vi "EOL CAN_Get_Motor_DTC's (2).vi"(10 "DTC Select Array":bool[](array[boolean])=[FALSE, FALSE, FALSE, FALSE, FALSE, FALSE, FALSE, FALSE, FALSE, FALSE, FALSE, FALSE, FALSE, FALSE, FALSE, FALSE, FALSE, FALSE, FALSE, FALSE], 11 "NetworkObjHandle":u32) -> (0 "DTC's Set":bool, 1 "DTC String":string, 2 "No. of DTC's":i32, 3 "Response Good?":bool, 5 "TxRx Data":string[][](array[string]))   [LabVIEW 2012]
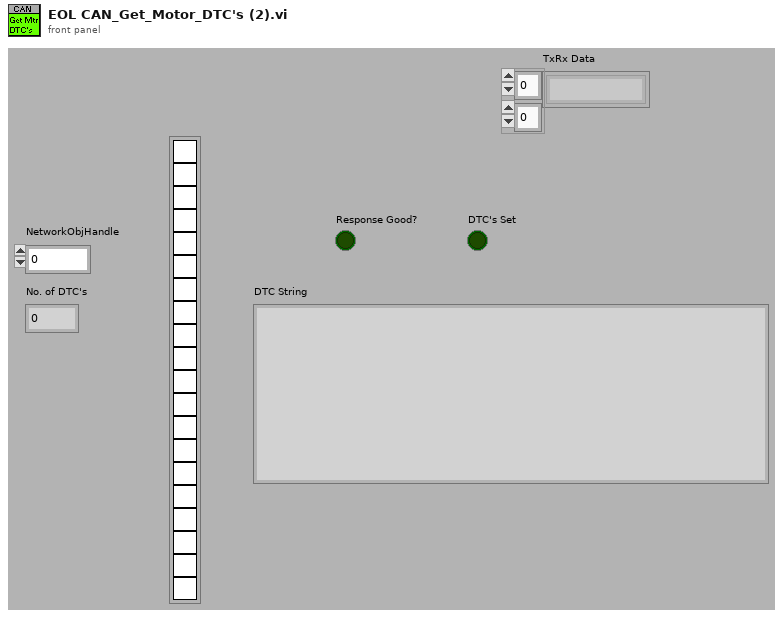
[diagram p1: front panel]
types:
  T1 = cluster{"Retry Counter":i32, "Array 1":u8[], "Array 21":u8[], "Array 22":u8[], "Array 23":u8[], "DTC's Array":u8[][], "No. of DTC's":i32, "Response Good?":bool, "TxRx Data":string[][]}
  T2 = typedef "xobjhandle.ctl" = u32
  T3 = typedef "CanFrameTimed.ctl" = cluster{"Timestamp":dbl, "ArbitrationId":u32, "IsRemote":u8, "DataLength":u8, "Data":u8[]}
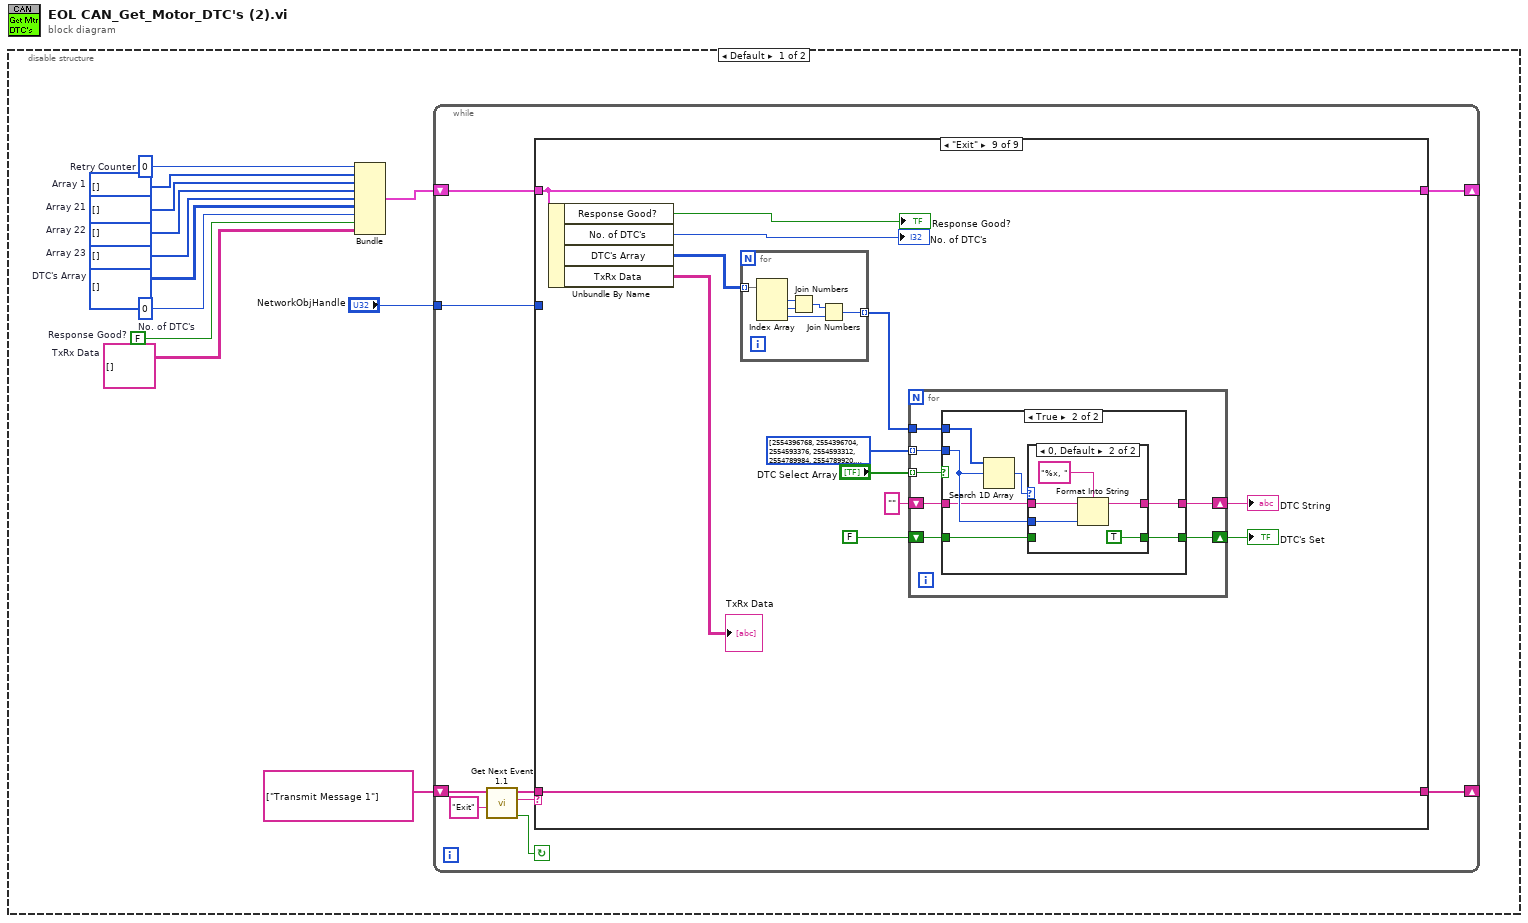
[diagram p0: block diagram]
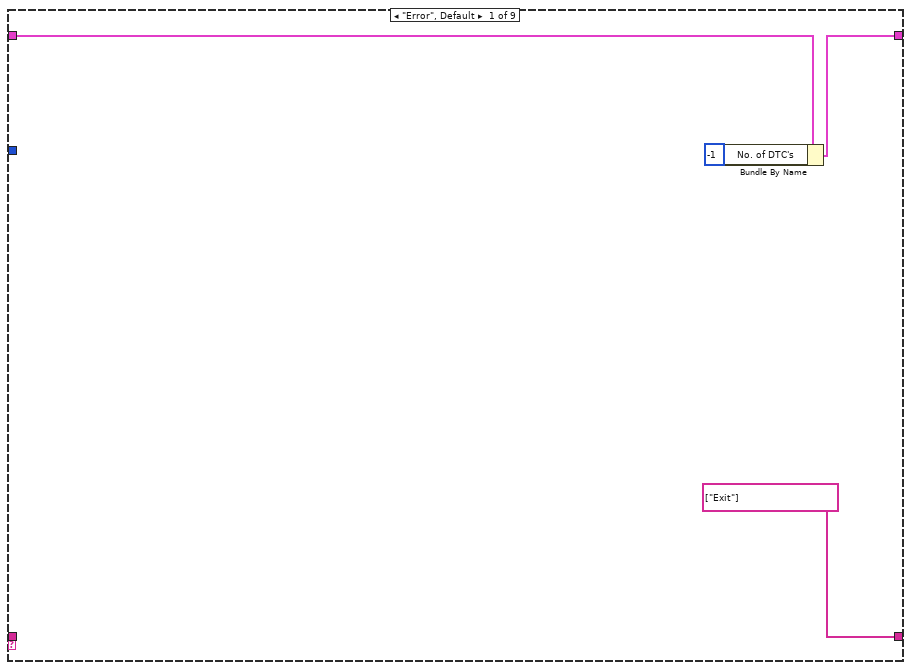
[diagram p2: hidden frame]
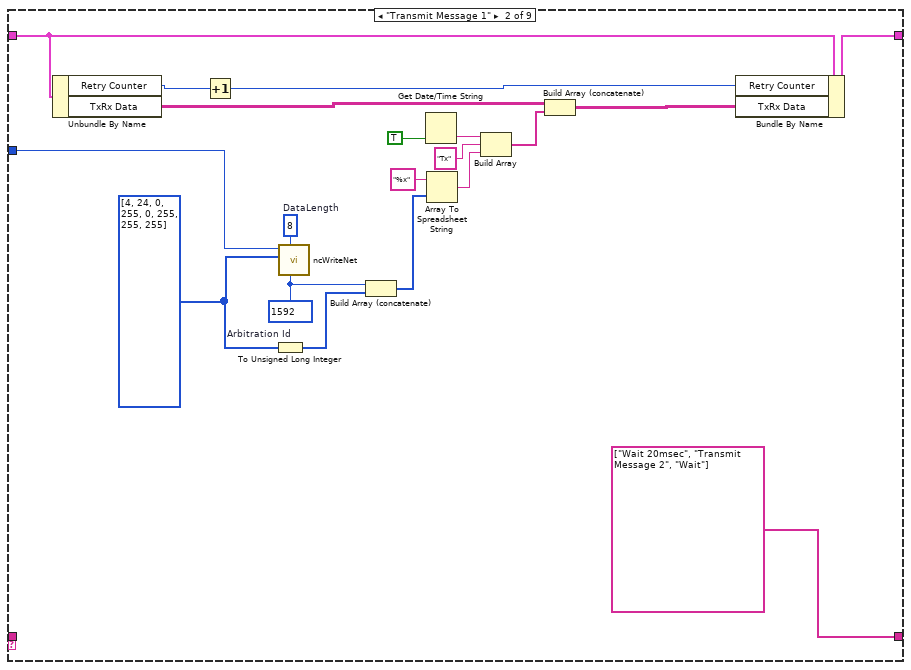
[diagram p3: hidden frame]
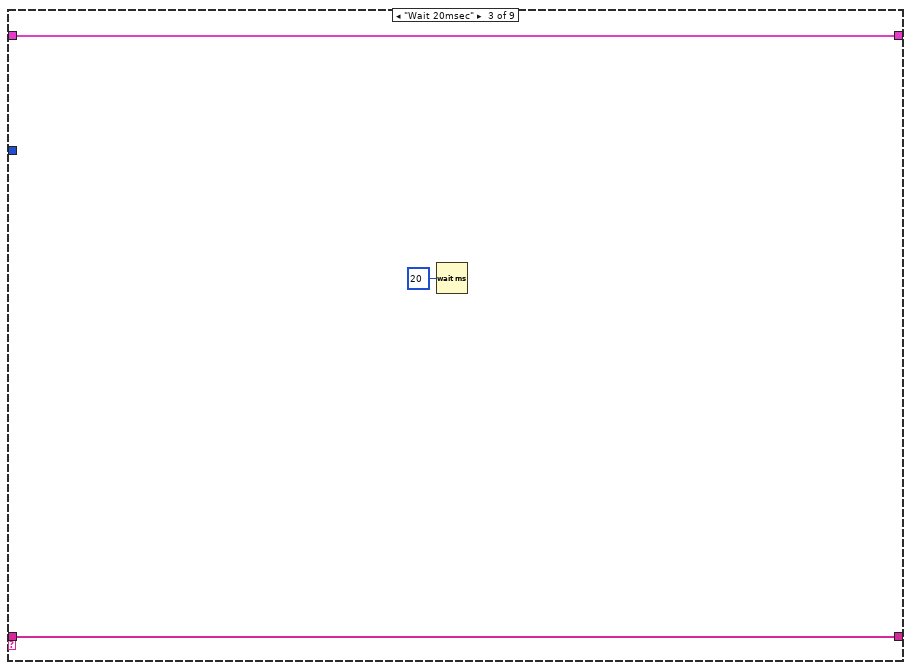
[diagram p4: hidden frame]
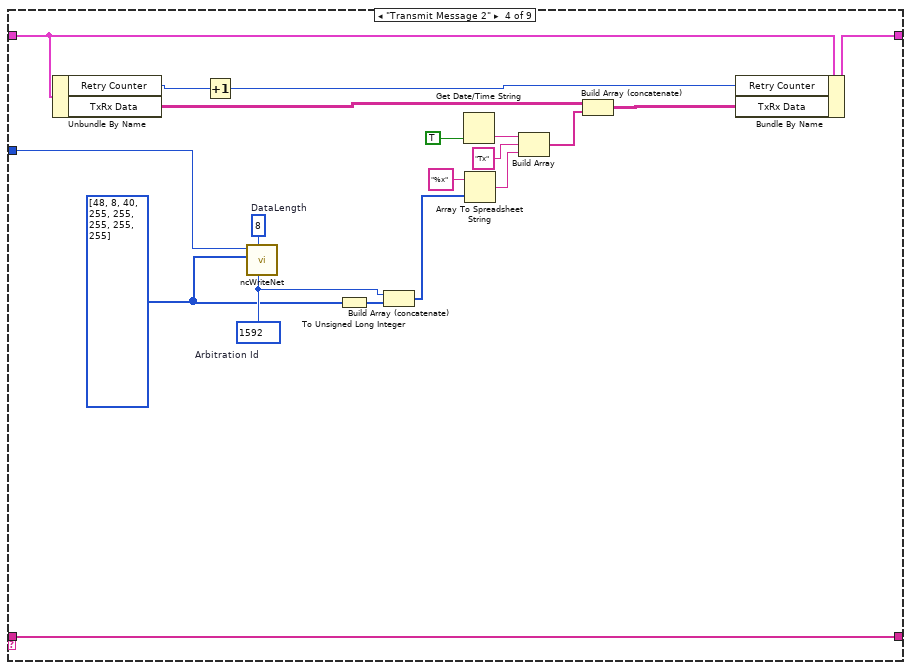
[diagram p5: hidden frame]
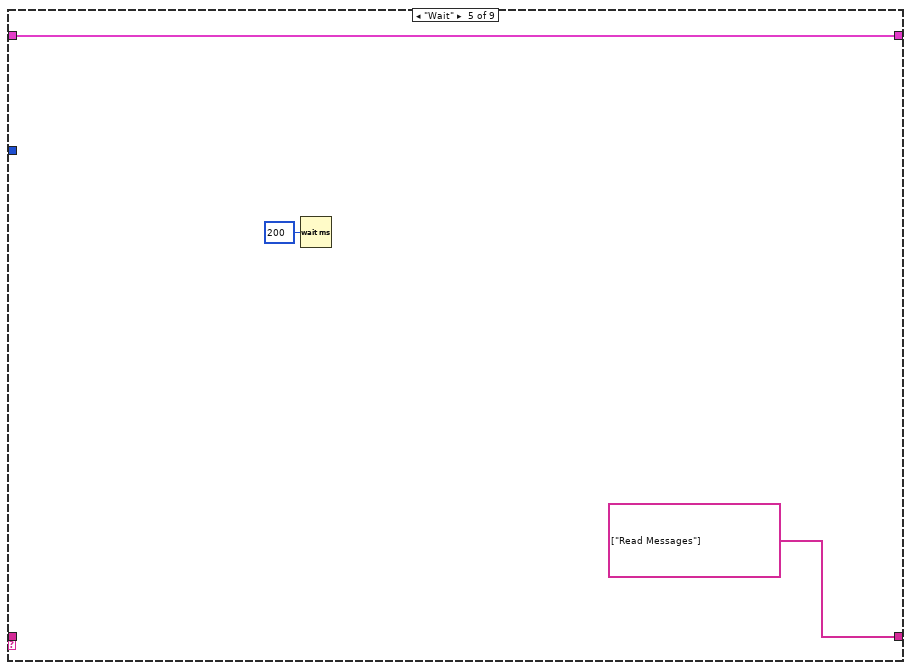
[diagram p6: hidden frame]
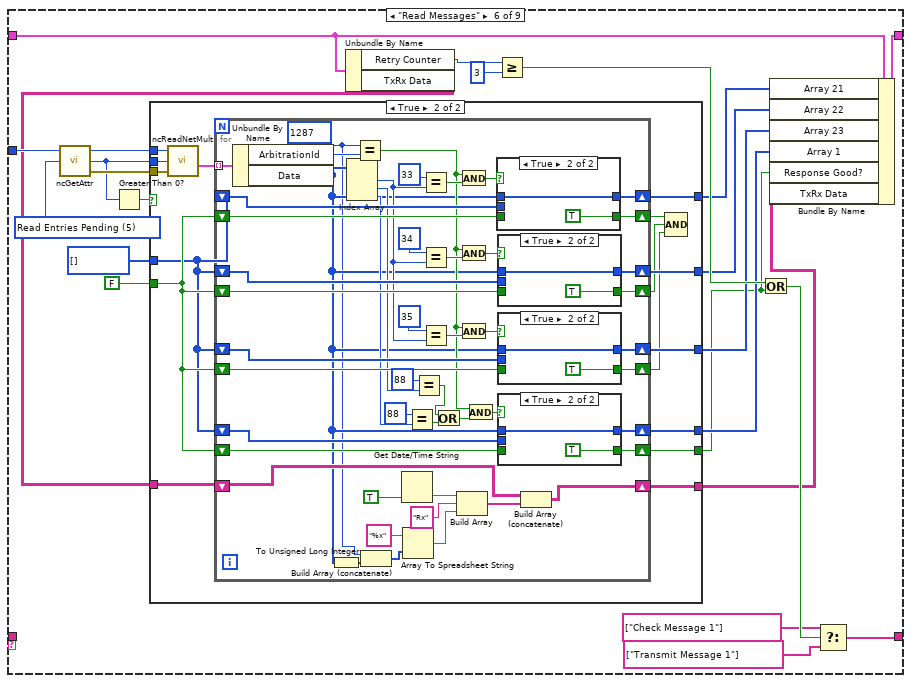
[diagram p7: hidden frame]
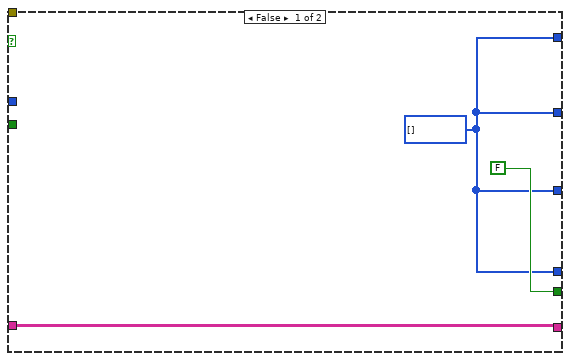
[diagram p8: hidden frame]
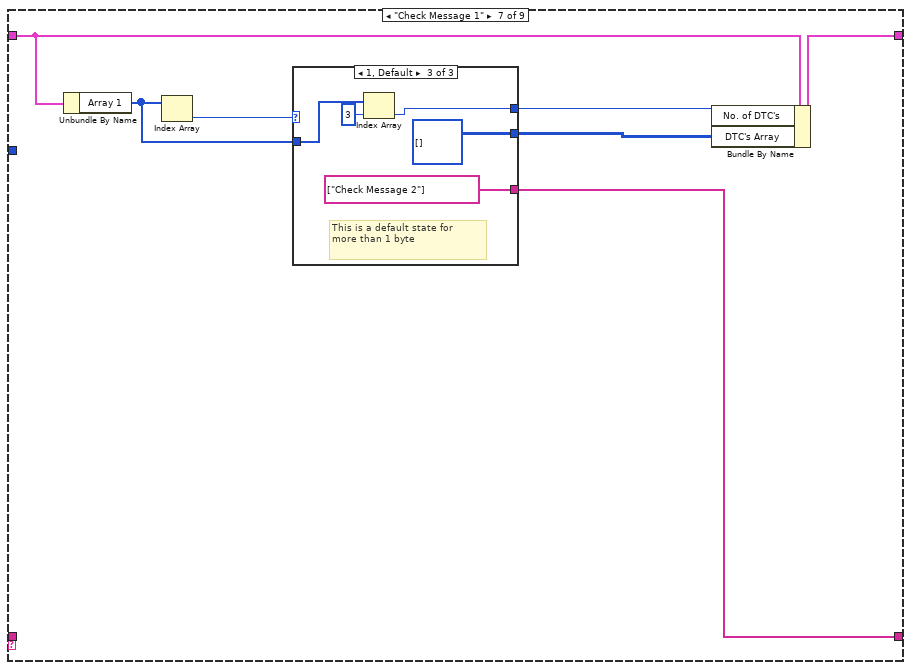
[diagram p13: hidden frame]
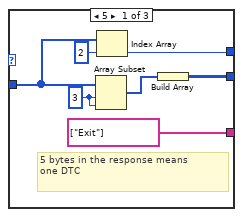
[diagram p14: hidden frame]
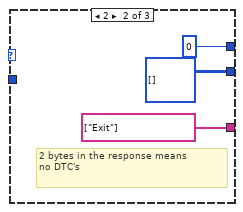
[diagram p15: hidden frame]
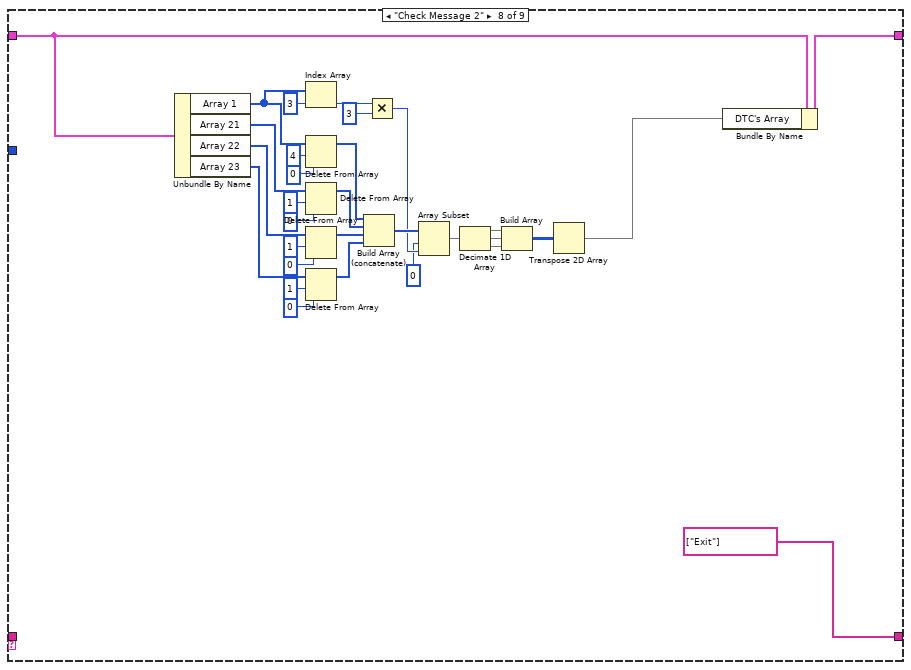
[diagram p16: hidden frame]
diagram:
  n1 = disable-structure shown="Default" {
    frame condition #0 (active) {
      w1 = string[][] []  # TxRx Data
      w2 = FALSE  # Response Good?
      w3 = 0  # No. of DTC's
      w4 = u8[][] []  # DTC's Array
      w5 = u8[] []  # Array 1
      w6 = u8[] []  # Array 23
      w7 = u8[] []  # Array 22
      w8 = u8[] []  # Array 21
      w10 = 0  # Retry Counter
      n2 = Bundle("Retry Counter"=w10, "Array 1"=w5, "Array 21"=w8, "Array 22"=w7, "Array 23"=w6, "DTC's Array"=w4, "No. of DTC's"=w3, "Response Good?"=w2, "TxRx Data"=w1) -> (w9:T1)  [unwired: 1 in]
      n3 = while {
        shift-right: [w18] -> _
        shift-left: string[] ["Transmit Message 1"] ("event queue out") -> [w17]
        tunnel: "NetworkObjHandle" -> [w16]
        shift-right: [w14] -> _
        shift-left: w9 -> [w15]
        stop <- w21 continue-if-true
        n4 = call "Get Next Event 1.1.vi"("Exit Event"="Exit", "event queue in"=w17) -> ("Condition (Exit:F)"=w21:bool, "next event"=w20:string, "event queue out"=w19:string[])  [unwired: 6 in, 1 out]
        n5 = case shown="\"Exit\"" w20 {
          tunnel: w19 -> [_ _ w46 w61 _ _ _ _ w243]
          tunnel: [string[] ["Exit"] ("event queue out") string[] ["Wait 20msec", "Transmit Message 2", "Wait"] ("event queue out") w46 w61 string[] ["Read Messages"] ("event queue out") w77 w184 string[] ["Exit"] ("event queue out") w243] -> w18
          tunnel: w16 -> [_ w39 _ w62 _ w76 _ _ _]
          tunnel: w15 -> [w24 w43 w47 w65 w69 w79 w183 w215 w241]
          tunnel: [w23 w41 w47 w63 w69 w78 w182 w214 w241] -> w14
          frame "Error", Default {
            n6 = Bundle By Name(cluster=w24, "No. of DTC's"=-1) -> (w23:T1)
          }
          frame "Transmit Message 1" {
            w37 = u32 1592  # Arbitration Id
            w38 = u32 8  # DataLength
            w36 = u8[] [4, 24, 0, 255, 0, 255, 255, 255] ("Transmit Data")
            n7 = Unbundle By Name(w43) -> ("Retry Counter"=w44:i32, "TxRx Data"=w27:string[][])
            n8 = Increment(x=w44) -> (x+1=w42:i32)
            n9 = To Unsigned Long Integer(number=w36) -> (unsigned 32bit integer=w29:u32[])
            n10 = call <vilib>:"ncWriteNet.vi"("ArbitrationId"=w37, "DataLength"=w38, "Data"=w36, "ObjHandle in"=w39) -> ()  [unwired: 2 in, 2 out]
            n11 = Build Array (concatenate)(w37, w29) -> (w28:u32[])
            n12 = Get Date/Time String(want seconds? (F)=TRUE) -> (time string=w32:string)  [unwired: 2 in, 1 out]
            n13 = Array To Spreadsheet String(array=w28, 3:"%x" ("format string")) -> (spreadsheet string=w34:string)  [unwired: 1 in]
            n14 = Build Array(w32, "Tx" ("format string"), w34) -> (w35:string[])
            n15 = Build Array (concatenate)(w27, w35) -> (w26:string[][])
            n16 = Bundle By Name(cluster=w43, "Retry Counter"=w42, "TxRx Data"=w26) -> (w41:T1)
          }
          frame "Wait 20msec" {
            n17 = Wait (ms)(milliseconds to wait=u32 20) -> ()  [unwired: 1 out]
          }
          frame "Transmit Message 2" {
            w59 = u32 1592  # Arbitration Id
            w60 = u32 8  # DataLength
            w58 = u8[] [48, 8, 40, 255, 255, 255, 255, 255] ("Transmit Data")
            n18 = Unbundle By Name(w65) -> ("Retry Counter"=w66:i32, "TxRx Data"=w48:string[][])
            n19 = Increment(x=w66) -> (x+1=w64:i32)
            n20 = call <vilib>:"ncWriteNet.vi"("ArbitrationId"=w59, "DataLength"=w60, "Data"=w58, "ObjHandle in"=w62) -> ()  [unwired: 2 in, 2 out]
            n21 = To Unsigned Long Integer(number=w58) -> (unsigned 32bit integer=w57:u32[])
            n22 = Build Array (concatenate)(w59, w57) -> (w49:u32[])
            n23 = Get Date/Time String(want seconds? (F)=TRUE) -> (time string=w53:string)  [unwired: 2 in, 1 out]
            n24 = Array To Spreadsheet String(array=w49, 3:"%x" ("format string")) -> (spreadsheet string=w55:string)  [unwired: 1 in]
            n25 = Build Array(w53, "Tx" ("format string"), w55) -> (w56:string[])
            n26 = Build Array (concatenate)(w48, w56) -> (w50:string[][])
            n27 = Bundle By Name(cluster=w65, "Retry Counter"=w64, "TxRx Data"=w50) -> (w63:T1)
          }
          frame "Wait" {
            n28 = Wait (ms)(milliseconds to wait=u32 200) -> ()  [unwired: 1 out]
          }
          frame "Read Messages" {
            w91 = u32 5 items=["(reserved)", "Protocol Version", "Software Version", "Object State", "(reserved)", "Read Entries Pending", "Write Entries Pending", "ReadMult Size for Notification", "Listen Only?", "Self Reception?", "Transmit Error Counter", "Receive Error Counter", "Single Shot Transmit?", "Series 2 Filter Mode", "Series 2 Mask", "Series 2 Comparator", "Serial Number", "Form Factor", "Series", "Transceiver Type", "Interface Number", "Series 2 Error/Arb Capture", "Transceiver Mode", "Transceiver External Outputs", "Transceiver External Inputs", "Start Trigger Behavior", "Log Comm Warnings", "User RTSI Frame", "Transmit Mode", "Log Start Trigger?", "Timestamp Format", "Master Timebase Rate", "Virtual Bus Timing"] ("AttrId")
            n29 = call <vilib>:"ncGetAttr.vi"("AttrId"=w91, "ObjHandle in"=w76) -> ("Error out"=w93:errorcluster, "AttrValue"=w89:u32, "ObjHandle out"=w92:T2)  [unwired: 1 in]
            n30 = Greater Than 0?(x=w89) -> (x > 0?=w90:bool)
            n31 = Unbundle By Name(w79) -> ("Retry Counter"=w85:i32, "TxRx Data"=w71:string[][])
            n32 = case shown="True" w90 {
              tunnel: w89 -> [_ w112]
              tunnel: w93 -> [_ w111]
              tunnel: w92 -> [_ w110]
              tunnel: [FALSE w99] -> w72
              tunnel: [w95 w108] -> w84
              tunnel: u16[] [] ("Data Array") -> [_ w100]
              tunnel: FALSE -> [_ w101]
              tunnel: [w95 w106] -> w81
              tunnel: [w95 w104] -> w80
              tunnel: [w95 w102] -> w75
              tunnel: w71 -> [w94 w98]
              tunnel: [w94 w97] -> w70
              frame False {
                w95 = u16[] [] ("Data Array")
              }
              frame True {
                n33 = call <vilib>:"ncReadNetMult.vi"("ObjHandle in"=w110, "Requested Number of Frames"=w112, "Error in"=w111) -> ("Data"=w109:T3[])  [unwired: 3 out]
                n34 = for {
                  tunnel: w109 -> [w161] mode=indexing
                  shift-right: [w159] -> w108
                  shift-left: w100 -> [w158]
                  shift-right: [w157] -> w107
                  shift-left: w101 -> [w156]
                  shift-right: [w153] -> w105
                  shift-left: w101 -> [w146]
                  shift-right: [w152] -> w106
                  shift-left: w100 -> [w151]
                  shift-right: [w139] -> w103
                  shift-left: w101 -> [w145]
                  shift-right: [w140] -> w104
                  shift-left: w100 -> [w141]
                  shift-right: [w138] -> w99
                  shift-left: w101 -> [w133]
                  shift-right: [w137] -> w102
                  shift-left: w100 -> [w136]
                  shift-right: [w117] -> w97
                  shift-left: w98 -> [w118]
                  w113 = u32 1287 ("x")
                  n35 = Unbundle By Name(w161) -> ("ArbitrationId"=w160:u32, "Data"=w115:u8[])
                  n36 = To Unsigned Long Integer(number=w115) -> (unsigned 32bit integer=w114:u32[])
                  n37 = Index Array(array=w115) -> (element #1=w131:u8, element #2=w130:u8, element #3=w128:u8)  [unwired: 3 in]
                  n38 = Equal?(x=w113, y=w160) -> (x = y?=w132:bool)
                  n39 = Build Array (concatenate)(w113, w114) -> (w116:u32[])
                  n40 = Get Date/Time String(want seconds? (F)=TRUE) -> (time string=w121:string)  [unwired: 2 in, 1 out]
                  n41 = Array To Spreadsheet String(array=w116, 3:"%x" ("format string")) -> (spreadsheet string=w123:string)  [unwired: 1 in]
                  n42 = Equal?(x=u16 88 ("y"), y=w128) -> (x = y?=w126:bool)
                  n43 = Equal?(x=u16 88 ("y"), y=w130) -> (x = y?=w127:bool)
                  n44 = Equal?(x=u16 33 ("y"), y=w131) -> (x = y?=w154:bool)
                  n45 = Equal?(x=u16 34 ("y"), y=w131) -> (x = y?=w150:bool)
                  n46 = Equal?(x=u16 35 ("y"), y=w131) -> (x = y?=w142:bool)
                  n47 = Or(x=w127, y=w126) -> (x .or. y?=w125:bool)
                  n48 = Build Array(w121, "Rx" ("format string"), w123) -> (w124:string[])
                  n49 = And(x=w132, y=w154) -> (x .and. y?=w155:bool)
                  n50 = And(x=w132, y=w150) -> (x .and. y?=w149:bool)
                  n51 = And(x=w132, y=w142) -> (x .and. y?=w143:bool)
                  n52 = And(x=w132, y=w125) -> (x .and. y?=w135:bool)
                  n53 = case shown="True" w155 {
                    tunnel: w115 -> [_ w176]
                    tunnel: [w175 w176] -> w159
                    tunnel: w158 -> [w175 _]
                    tunnel: [w174 TRUE] -> w157
                    tunnel: w156 -> [w174 _]
                    frame False {
                    }
                    frame True {
                    }
                  }
                  n54 = case shown="True" w149 {
                    tunnel: w115 -> [_ w172]
                    tunnel: [w171 w172] -> w152
                    tunnel: w151 -> [w171 _]
                    tunnel: [w170 TRUE] -> w153
                    tunnel: w146 -> [w170 _]
                    frame False {
                    }
                    frame True {
                    }
                  }
                  n55 = case shown="True" w143 {
                    tunnel: w115 -> [_ w168]
                    tunnel: [w167 w168] -> w140
                    tunnel: w141 -> [w167 _]
                    tunnel: [w166 TRUE] -> w139
                    tunnel: w145 -> [w166 _]
                    frame False {
                    }
                    frame True {
                    }
                  }
                  n56 = case shown="True" w135 {
                    tunnel: w115 -> [_ w164]
                    tunnel: [w163 w164] -> w137
                    tunnel: w136 -> [w163 _]
                    tunnel: [w162 TRUE] -> w138
                    tunnel: w133 -> [w162 _]
                    frame False {
                    }
                    frame True {
                    }
                  }
                  n57 = Build Array (concatenate)(w118, w124) -> (w117:string[][])
                }
                n58 = Compound Arithmetic op=AND(w107, w105, w103) -> ()  [unwired: 1 out]
              }
            }
            n59 = Greater Or Equal?(x=w85, y=3) -> (x >= y?=w87:bool)
            n60 = Or(x=w87, y=w72) -> (x .or. y?=w86:bool)
            n61 = Bundle By Name(cluster=w79, "Array 21"=w84, "Array 22"=w81, "Array 23"=w80, "Array 1"=w75, "Response Good?"=w72, "TxRx Data"=w70) -> (w78:T1)
            n62 = Select(t=string[] ["Check Message 1"] ("f"), s=w86, f=string[] ["Transmit Message 1"] ("event queue out")) -> (s? t:f=w77:string[])
          }
          frame "Check Message 1" {
            n63 = Unbundle By Name(w183) -> ("Array 1"=w179:u8[])
            n64 = Index Array(array=w179) -> (element=w180:u8)  [unwired: 1 in]
            n65 = case shown="1, Default" w180 {
              tunnel: [string[] ["Exit"] ("event queue out") string[] ["Exit"] ("event queue out") string[] ["Check Message 2"] ("event queue out")] -> w184
              tunnel: [w189 u16[][] [] u16[][] []] -> w181
              tunnel: w179 -> [w186 _ w197]
              tunnel: [w185 u16 0 ("Motor Temperature") w195] -> w178
              frame 5 {
                w188 = 3 ("index")
                # "5 bytes in the response means\none DTC"
                n66 = Array Subset(array=w186, index=w188, length=w188) -> (w190:u8[])
                n67 = Index Array(array=w186, index=2) -> (element=w185:u8)
                n68 = Build Array(w190) -> (w189:u8[][])
              }
              frame 2 {
                # "2 bytes in the response means\nno DTC's"
              }
              frame 1, Default {
                # "This is a default state for \nmore than 1 byte"
                n69 = Index Array(array=w197, index=3) -> (element=w195:u8)
              }
            }
            n70 = Bundle By Name(cluster=w183, "No. of DTC's"=w178, "DTC's Array"=w181) -> (w182:T1)
          }
          frame "Check Message 2" {
            n71 = Unbundle By Name(w215) -> ("Array 1"=w211:u8[], "Array 21"=w230:u8[], "Array 22"=w229:u8[], "Array 23"=w228:u8[])
            n72 = Index Array(array=w211, index=3) -> (element=w223:u8)
            n73 = Delete From Array(array=w211, length=4 ("index"), index=0) -> (array with subset deleted=w210:u8[])  [unwired: 1 out]
            n74 = Delete From Array(array=w230, length=1, index=0) -> (array with subset deleted=w226:u8[])  [unwired: 1 out]
            n75 = Delete From Array(array=w229, length=1, index=0) -> (array with subset deleted=w225:u8[])  [unwired: 1 out]
            n76 = Delete From Array(array=w228, length=1, index=0) -> (array with subset deleted=w224:u8[])  [unwired: 1 out]
            n77 = Build Array (concatenate)(w210, w226, w225, w224) -> (w222:u8[])
            n78 = Multiply(x=w223, y=u16 3) -> (x*y=w221:u16)
            n79 = Array Subset(array=w222, index=0, length=w221) -> (w219:u8[])
            n80 = Decimate 1D Array(w219) -> (w218:u8[], w217:u8[], w216:u8[])
            n81 = Build Array(w218, w217, w216) -> (w213:u8[][])
            n82 = Transpose 2D Array(2D array=w213) -> (transposed array=w200:u8[][])
            n83 = Bundle By Name(cluster=w215, "DTC's Array"=w200) -> (w214:T1)
          }
          frame "Exit" {
            n84 = Unbundle By Name(w241) -> ("Response Good?"=→"Response Good?":bool, "No. of DTC's"=→"No. of DTC's":i32, "DTC's Array"=w242:u8[][], "TxRx Data"=→"TxRx Data":string[][])
            n85 = for {
              tunnel: w242 -> [w272] mode=indexing
              tunnel: [w267] -> w235 mode=indexing
              n86 = Index Array(array=w272) -> (element #1=w270:u8, element #2=w271:u8, element #3=w268:u8)  [unwired: 3 in]
              n87 = Join Numbers(hi=w270, lo=w271) -> ((hi.lo)=w269:u16)
              n88 = Join Numbers(hi=w269, lo=w268) -> ((hi.lo)=w267:u32)
            }
            n89 = for {
              tunnel: u32[] [2554396768, 2554396704, 2554593376, 2554593312, 2554789984, 2554789920, 2554921056, 2554789920, 2701983840, 2701983776, 2702049376, 2702049312, 2720464992, 2720464928, 3222863968, 3222863904, 3242262624, 3242262560, 3243573344, 3243573280] ("Array") -> [w249] mode=indexing
              tunnel: "DTC Select Array" -> [w250] mode=indexing
              tunnel: w235 -> [w248]
              shift-right: [w247] -> w237
              shift-left: "" -> [w246]
              shift-right: [w244] -> w232
              shift-left: FALSE -> [w245]
              n90 = case shown="True" w250 {
                tunnel: w249 -> [_ w258]
                tunnel: w248 -> [_ w259]
                tunnel: [w252 w257] -> w247
                tunnel: w246 -> [w252 w256]
                tunnel: w245 -> [w251 w254]
                tunnel: [w251 w253] -> w244
                frame False {
                }
                frame True {
                  n91 = Search 1D Array(1D array=w259, element=w258) -> (index of element=w255:i32)  [unwired: 1 in]
                  n92 = case shown="0, Default" w255 {
                    tunnel: w258 -> [_ w266]
                    tunnel: [w261 w264] -> w257
                    tunnel: w256 -> [w261 w263]
                    tunnel: w254 -> [w260 _]
                    tunnel: [w260 TRUE] -> w253
                    frame -1 {
                    }
                    frame 0, Default {
                      n93 = Format Into String(format string="%x, ", initial string=w263, w266) -> (resulting string=w264:string)  [unwired: 1 in, 1 out]
                    }
                  }
                }
              }
            }
            "DTC's Set" <- w232
            "DTC String" <- w237
          }
        }
      }
    }
    frame condition #1 {
    }
  }
